vi "ArrayConstant.vi"() -> (0 "VCI_CAN_OBJ_RN":T1(array[cluster]))   [LabVIEW 2013]
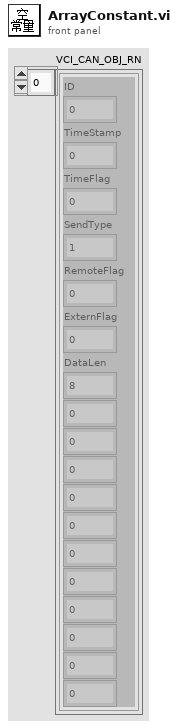
[diagram p1: front panel]
types:
  T1 = cluster{"ID":u32, "TimeStamp":u32, "TimeFlag":u8, "SendType":u8, "RemoteFlag":u8, "ExternFlag":u8, "DataLen":u8, u8, u8, u8, u8, u8, u8, u8, u8, u8, u8, u8}[]
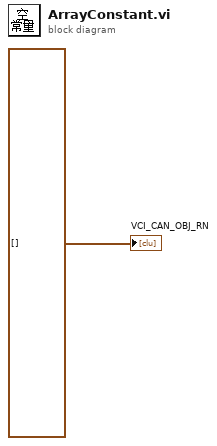
[diagram p0: block diagram]
diagram:
  "VCI_CAN_OBJ_RN" <- T1 [] ("VCI_CAN_OBJ_RN")
